vi "SmartMotor Initialize Chain.vi"(0 "reference in":refnum<class "SmartMotor.lvclass">, 5 "SmartMotor Chain VISA Resource":refnum<visa-resource-name>, 7 "Number of Motors In Motor Chain":i32 min=0 max=10 step=1, 11 "Error In":errorcluster) -> (4 "reference out":refnum<class "SmartMotor.lvclass">, 6 "SmartMotor Chain VISA Session":refnum<visa-resource-name>, 15 "Error Out":errorcluster)   [LabVIEW 2017, in "SmartMotor.lvclass"]
uses:
  SmartMotor.lvclass
  <vilib>/Instr/_visa.llb/VISA Open Access Mode.ctl
  <vilib>/Instr/_visa.llb/VISA Configure Serial Port (Instr).vi
panel:
  in  "Computer COM Port Name (Allias)":string
  out "Sample Read Output":string
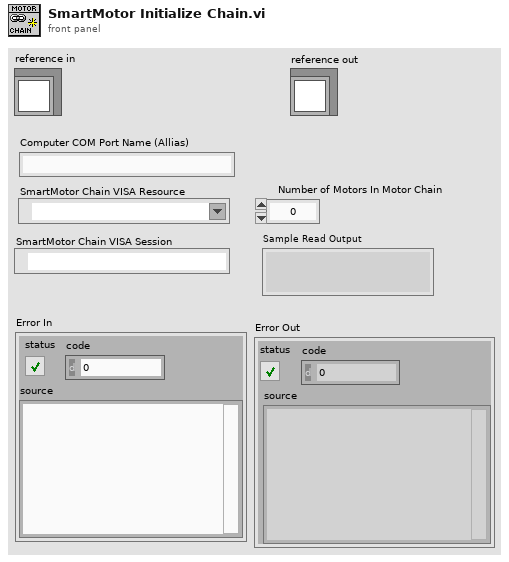
[diagram p1: front panel]
types:
  T1 = typedef "VISA Open Access Mode.ctl" = u32
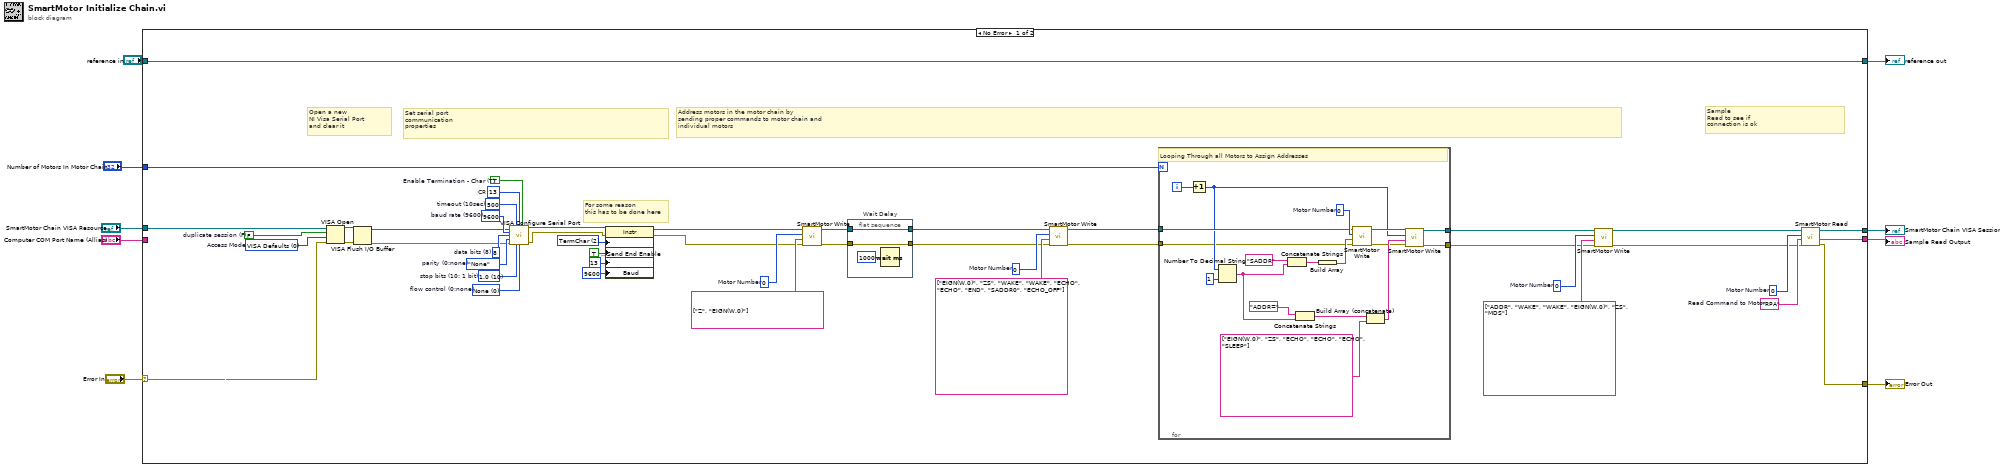
[diagram p0: block diagram]
diagram:
  n1 = case shown="No Error" "Error In" {
    selector: "Error In" -> [w49 w78]
    tunnel: "Number of Motors In Motor Chain" -> [w52 _]
    tunnel: [w10 w78] -> w8
    tunnel: [w47 _] -> w7
    tunnel: "reference in" -> [w48 w79]
    tunnel: [w48 w79] -> w4
    tunnel: [w46 _] -> w3
    tunnel: "Computer COM Port Name (Allias)" -> [_ _]
    tunnel: "SmartMotor Chain VISA Resource" -> [w45 _]
    frame No Error {
      w26 = u8 0  # Motor Number
      w30 = u16 2 items=["None", "LastBit", "TermChar", "Break"] ("Serial Settings:Serial End Mode for Writes")
      w36 = u16 0 items=["None", "XON/XOFF", "RTS/CTS", "XON/XOFF & RTS/CTS", "DTR/DSR", "XON/XOFF & DTR/DSR"]  # flow control (0:none)
      w37 = u16 10 items=["1.0"=10, "1.5"=15, "2.0"=20]  # stop bits (10: 1 bit)
      w38 = enum16{"None", "Odd", "Even", "Mark", "Space"}."None"  # parity (0:none)
      w39 = u16 8  # data bits (8)
      w40 = FALSE  # duplicate session (F)
      w41 = T1 0 items=["VISA Defaults"=0, "Exclusive Lock"=1, "Load Configured Settings"=4]  # Access Mode
      w42 = "RPA"  # Read Command to Motor
      w43 = 0  # Motor Number
      w50 = u32 9600  # baud rate (9600)
      w53 = u8 0  # Motor Number
      w54 = u8 0  # Motor Number
      w55 = TRUE  # Enable Termination - Char (T)
      w56 = u32 500  # timeout (10sec)
      # "CR"
      # "For some reason\nthis has to be done here"
      # "Sample\nRead to see if \nconnection is ok"
      # "Address motors in the motor chain by \nsending proper commands to motor chain and \nindividual motors"
      # "Set serial port\ncommunication \nproperties"
      # "Open a new\nNI Visa Serial Port\nand clear it"
      n2 = VISA Open(duplicate session (F)=w40, access mode=w41, error in (no error)=w49, VISA resource name=w45) -> (VISA resource name=w34:refnum<visa-resource-name>, error out=w19:errorcluster)  [unwired: 1 in]
      n3 = VISA Flush I/O Buffer(VISA resource name=w34, error in (no error)=w19) -> (VISA resource name out=w33:refnum<visa-resource-name>, error out=w18:errorcluster)  [unwired: 1 in]
      n4 = call-poly "VISA Configure Serial Port"("VISA resource name"=w33, "timeout (10sec)"=w56, "termination char\n(0xA = '\\n' = LF)"=u8 13 ("Message Based Settings:Termination Character"), "Enable Termination\nChar (T)"=w55, "baud rate (9600)"=w50, "data bits (8)"=w39, "parity (0:none)"=w38, "error in (no error)"=w18, "stop bits (10: 1 bit)"=w37, "flow control (0:none)"=w36) -> ("VISA resource name out"=w28:refnum<visa-resource-name>, "error out"=w17:errorcluster)  [unwired: 4 out]
      n5 = property class="Instr"(reference=w28, error in=w17, "Serial Settings:End Mode for Writes"=w30, "Message Based Settings:Send End Enable"=TRUE, "Message Based Settings:Termination Character"=u8 13, "Baud"=u32 9600 ("Serial Settings:Baud Rate")) -> (reference out=w27:refnum<visa-resource-name>, error out=w16:errorcluster)
      n6 = call "SmartMotor Write.vi"("VISA resource IN"=w27, "Motor Number"=w54, "Motor Command Array"=string[] ["Z", "EIGN(W,0)"], "Error In"=w16) -> ("VISA resource OUT"=w23:refnum<visa-resource-name>, "Error Out"=w15:errorcluster)  [unwired: 3 in, 1 out]
      n7 = flat-sequence "Wait Delay" {
        tunnel: w23 -> [w59]
        tunnel: [w59] -> w22
        tunnel: w15 -> [w57]
        tunnel: [w57] -> w14
        frame #0 {
          n8 = Wait (ms)(milliseconds to wait=u32 1000) -> ()  [unwired: 1 out]
        }
      }
      n9 = call "SmartMotor Write.vi"("VISA resource IN"=w22, "Motor Number"=w26, "Motor Command Array"=string[] ["EIGN(W,0)", "ZS", "WAKE", "WAKE", "ECHO", "ECHO", "END", "SADDR0", "ECHO_OFF"], "Error In"=w14) -> ("VISA resource OUT"=w25:refnum<visa-resource-name>, "Error Out"=w13:errorcluster)  [unwired: 3 in, 1 out]
      n10 = for {
        N: w52 -> [_]
        tunnel: w25 -> [w71]
        tunnel: [w65] -> w51
        tunnel: w13 -> [w60]
        tunnel: [w61] -> w12
        i -> [w70]
        w75 = u8 0  # Motor Number
        # "Looping Through all Motors to Assign Addresses"
        n11 = Increment(x=w70) -> (x+1=w69:i32)
        n12 = Number To Decimal String(number=w69, width (-)=i16 1) -> (decimal integer string=w66:string)
        n13 = Concatenate Strings("SADDR", w66) -> (w73:string)
        n14 = Concatenate Strings("ADDR=", w66) -> (w68:string)
        n15 = Build Array(w73) -> (w77:string[])
        n16 = call "SmartMotor Write.vi"("VISA resource IN"=w71, "Motor Number"=w75, "Motor Command Array"=w77, "Error In"=w60) -> ("VISA resource OUT"=w76:refnum<visa-resource-name>, "Error Out"=w62:errorcluster)  [unwired: 3 in, 1 out]
        n17 = Build Array (concatenate)(w68, string[] ["EIGN(W,0)", "ZS", "ECHO", "ECHO", "ECHO", "SLEEP"]) -> (w64:string[])
        n18 = call "SmartMotor Write.vi"("VISA resource IN"=w76, "Motor Number"=w69, "Motor Command Array"=w64, "Error In"=w62) -> ("VISA resource OUT"=w65:refnum<visa-resource-name>, "Error Out"=w61:errorcluster)  [unwired: 3 in, 1 out]
      }
      n19 = call "SmartMotor Write.vi"("VISA resource IN"=w51, "Motor Number"=w53, "Motor Command Array"=string[] ["ADDR", "WAKE", "WAKE", "EIGN(W,0)", "ZS", "MDS"], "Error In"=w12) -> ("VISA resource OUT"=w44:refnum<visa-resource-name>, "Error Out"=w11:errorcluster)  [unwired: 3 in, 1 out]
      n20 = call "SmartMotor Read.vi"("VISA resource IN"=w44, "Motor Number"=w43, "Read Command to Motor"=w42, "Error In"=w11) -> ("VISA resource OUT"=w47:refnum<visa-resource-name>, "Response From Motor"=w46:string, "Error Out"=w10:errorcluster)  [unwired: 1 in, 2 out]
    }
    frame Error {
    }
  }
  "SmartMotor Chain VISA Session" <- w7
  "Error Out" <- w8
  "reference out" <- w4
  "Sample Read Output" <- w3
